vi "Tiles and Channels.vi"(8 "error in (no error)":errorcluster, 10 "Type":enum16{"ADC", "DAC"}(ring), 11 "RFSoC Driver in":refnum<class "RFSoC Driver.lvclass">) -> (0 "error out":errorcluster, 1 "Tiles and converters out":i32[][](array[numeric]), 2 "Channels out":i32[](array[numeric]), 3 "RFSoC Driver out":refnum<class "RFSoC Driver.lvclass">)   [LabVIEW 2019, in "RFSoC Driver.lvclass"]
uses:
  RFSoC Driver.lvclass
  RFSoC Driver.lvclass/RFSoC Driver.ctl
  Read ADC Channels.vi
  Read DAC Channels.vi
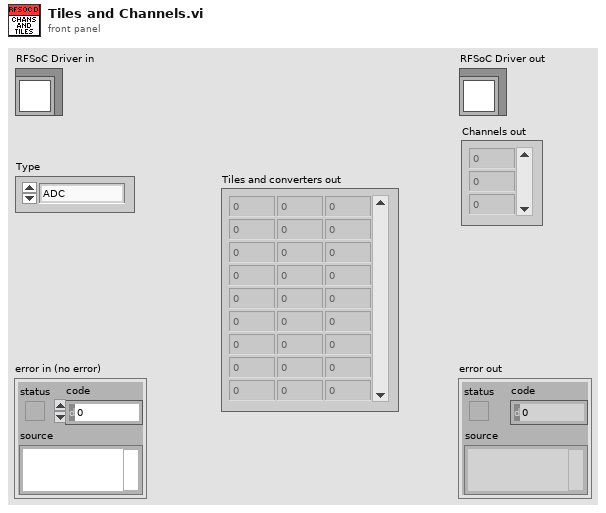
[diagram p1: front panel]
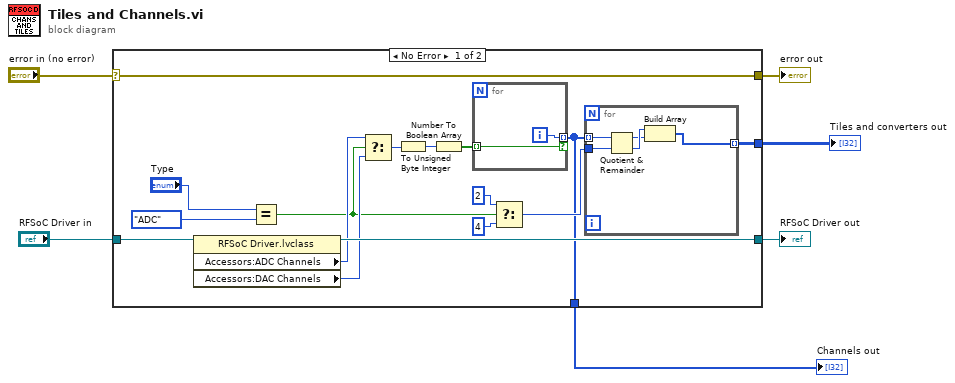
[diagram p0: block diagram]
diagram:
  n1 = case shown="No Error" "error in (no error)" {
    selector: "error in (no error)" -> [w22 w31]
    tunnel: [w22 w31] -> w5
    tunnel: [w21 w30] -> w3
    tunnel: "RFSoC Driver in" -> [w20 w30]
    tunnel: [w8 _] -> w2
    tunnel: [w7 _] -> w1
    frame No Error {
      n2 = property class="RFSoC Driver.lvclass"(reference=w20) -> (reference out=w21:refnum<class "RFSoC Driver.lvclass">, "Accessors:ADC Channels"=w17:i32, "Accessors:DAC Channels"=w16:i32)  [unwired: 1 in, 1 out]
      n3 = Equal?(x="Type", y=enum16{"ADC", "DAC"}."ADC") -> (x = y?=w10:bool)
      n4 = Select(t=w17, s=w10, f=w16) -> (s? t:f=w13:i32)
      n5 = To Unsigned Byte Integer(number=w13) -> (unsigned 8bit integer=w14:u8)
      n6 = Number To Boolean Array(number=w14) -> (Boolean array=w15:bool[])
      n7 = for {
        tunnel: w15 -> [w28] mode=indexing
        tunnel: [w29] -> w8 mode=indexing if=w28
        i -> [w29]
      }
      n8 = Select(t=2 ("y"), s=w10, f=4 ("y")) -> (s? t:f=w9:i32)
      n9 = for {
        tunnel: w9 -> [w25]
        tunnel: w8 -> [w24] mode=indexing
        tunnel: [w23] -> w7 mode=indexing
        n10 = Quotient & Remainder(x=w24, y=w25) -> (x-y*floor(x/y)=w26:i32, floor(x/y)=w27:i32)
        n11 = Build Array(w27, w26) -> (w23:i32[])
      }
    }
    frame Error {
    }
  }
  "error out" <- w5
  "RFSoC Driver out" <- w3
  "Channels out" <- w2
  "Tiles and converters out" <- w1
